vi "Get Routing Channel.vi"(8 "error in (no error)":errorcluster, 10 "Channel Ref":T4 format="%.0x", 11 "RAF Custom Device in":refnum<k24>) -> (0 "error out":errorcluster, 1 "Channel States":T1, 2 "Channel Name":string, 3 "RAF Custom Device out":refnum<k24>)   [LabVIEW 2017, in "Switch Scripting.lvlib"]
uses:
  Switch Scripting.lvlib
  NationalInstruments.VeriStand.SystemDefinitionAPI
  <vilib>/NI Veristand/Custom Device API/Custom Device Item Ref.ctl
  Channel States.ctl
  Routing State.ctl
  Connection.ctl
  <vilib>/NI Veristand/Custom Device API/Get Item Property (String).vi
  <vilib>/NI VeriStand/Custom Device API/Custom Device API.lvlib
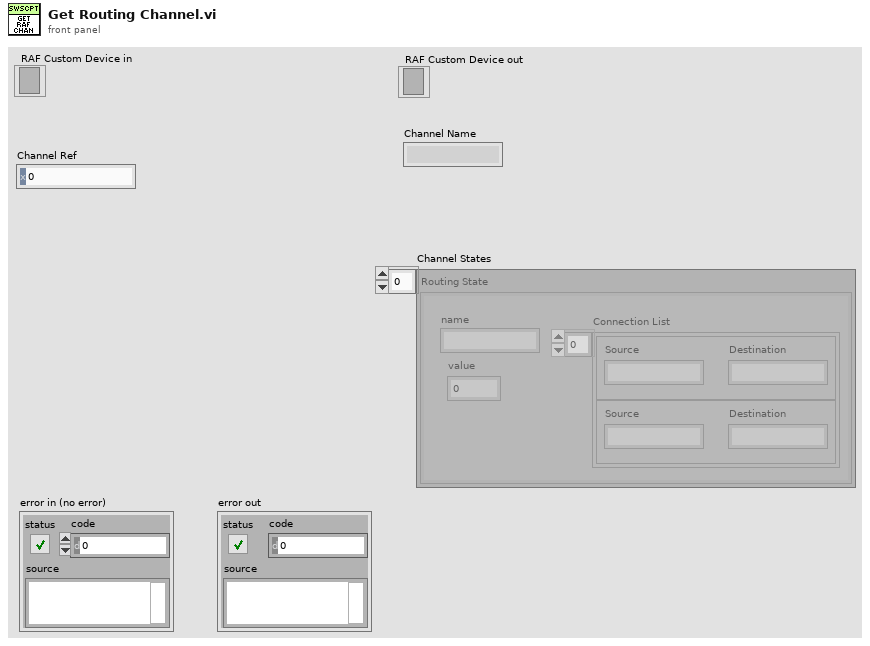
[diagram p1: front panel]
types:
  T1 = typedef "Switch Scripting.lvlib/Channel States.ctl" = T2[]
  T2 = typedef "Switch Scripting.lvlib/Routing State.ctl" = cluster{"name":string, "value":i32, "Connection List":T3[]}
  T3 = typedef "Switch Scripting.lvlib/Connection.ctl" = cluster{"Source":string, "Destination":string}
  T4 = typedef "Custom Device API.lvlib/Custom Device Item Ref.ctl" = u64
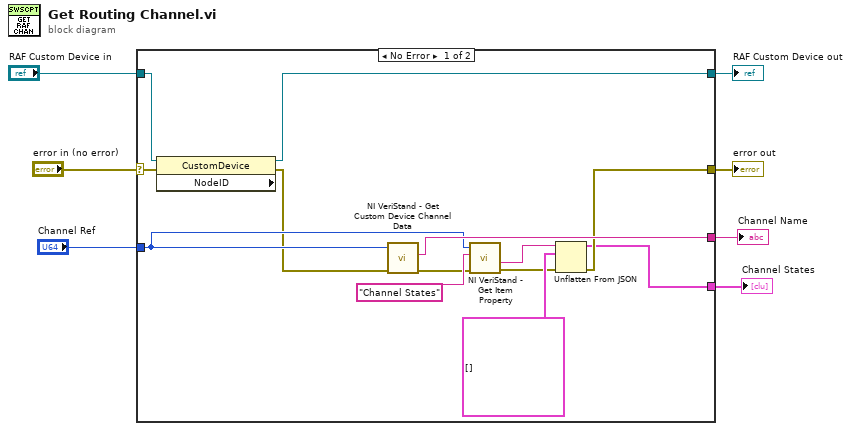
[diagram p0: block diagram]
diagram:
  n1 = case shown="No Error" "error in (no error)" {
    selector: "error in (no error)" -> [w19 w22]
    tunnel: [w9 w22] -> w7
    tunnel: [w20 w21] -> w6
    tunnel: "RAF Custom Device in" -> [w18 w21]
    tunnel: "Channel Ref" -> [w16 _]
    tunnel: [w17 _] -> w2
    tunnel: [w8 _] -> w1
    frame No Error {
      n2 = property class="CustomDevice" props=["NodeID"](reference=w18, error in=w19) -> (reference out=w20:refnum<k24>, error out=w14:errorcluster)  [unwired: 1 out]
      n3 = call <vilib>:"NI VeriStand - Get Custom Device Channel Data.vi"("error in (no error)"=w14, "Channel Ref in"=w16) -> ("error out"=w13:errorcluster, "Channel Name"=w17:string)  [unwired: 4 in, 4 out]
      n4 = call-poly <vilib>:"NI VeriStand - Get Item Property.vi"("error in (no error)"=w13, "Property Name"="Channel States" ("String"), "Item Ref in"=w16) -> ("error out"=w10:errorcluster, "Value"=w12:string)  [unwired: 5 in, 2 out]
      n5 = Unflatten From JSON(JSON string=w12, type and defaults=T1 [] ("Channel States"), error in (no error)=w10) -> (value=w8:T1, error out=w9:errorcluster)  [unwired: 4 in]
    }
    frame Error {
    }
  }
  "error out" <- w7
  "RAF Custom Device out" <- w6
  "Channel Name" <- w2
  "Channel States" <- w1
